vi "Server_Demo_VIs.vi"(11 "Only get This VIs path":bool) -> (3 "path":path)   [LabVIEW 2011]
doc: "reentrant"
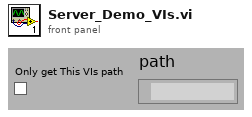
[diagram p1: front panel]
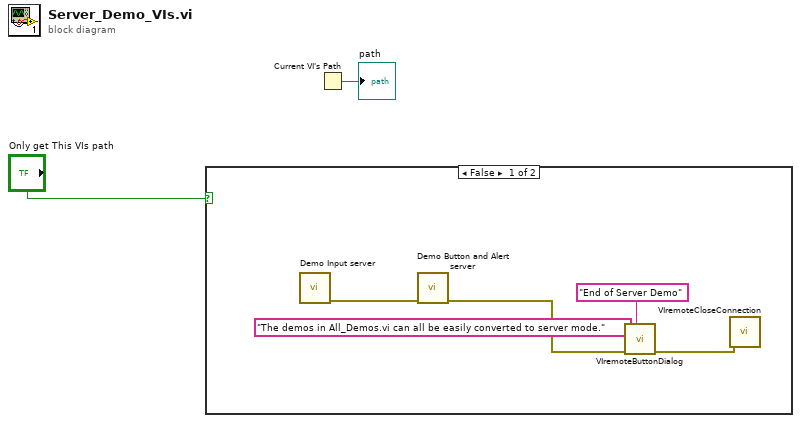
[diagram p0: block diagram]
diagram:
  n1 = case shown="False" "Only get This VIs path" {
    frame False {
      n2 = call "Demo Input server.vi"() -> ("error out"=w7:errorcluster)  [unwired: 1 in, 10 out]
      n3 = call "Demo Button and Alert server.vi"("error in (no error)"=w7) -> ("error out"=w6:errorcluster)  [unwired: 10 out]
      n4 = call "VIremoteButtonDialog.vi"("Window Title (\"\")"="End of Server Demo" ("Window Title (\"\")"), "error in (no error)"=w6, "message"="The demos in All_Demos.vi can all be easily converted to server mode.") -> ("error out"=w3:errorcluster)  [unwired: 1 in, 7 out]
      n5 = call "VIremoteCloseConnection.vi"("error in (no error)"=w3) -> ()  [unwired: 1 in, 10 out]
    }
    frame True {
    }
  }
  n6 = Current VI's Path() -> (path=→"path":path)
